vi "Update.vi"(8 "error in (no error)":errorcluster, 10 "Message in":refnum<class "UpdateMessage.lvclass">, 11 "AOTF in":refnum<class "Invivo_AOTF.lvclass">) -> (0 "error out":errorcluster, 3 "AOTF out":refnum<class "Invivo_AOTF.lvclass">)   [LabVIEW 2012, in "Invivo_AOTF.lvclass"]
doc: "The update method processes the command 'update'. \n\nThe command 'update' is used for receiving new values to be set to the private data of the class. This could be seen as a public set method for setting new parameters to the private class data."
uses:
  Invivo_AOTF.lvclass
  <vilib>/Distrio/Murmex/UpdateMessage/UpdateMessage.lvclass
  Invivo_AOTF.lvclass/Invivo_AOTF.ctl
  Controls/laser line enum.ctl
  <vilib>/Distrio/Murmex/Murmex/Murmex.lvclass
panel:
  # "This method is called when the UPDATE\ntrigger is sent. \n\nOverride this method when your component needs to\nrespond to this trigger. \n\nCall parent for proper implementation"
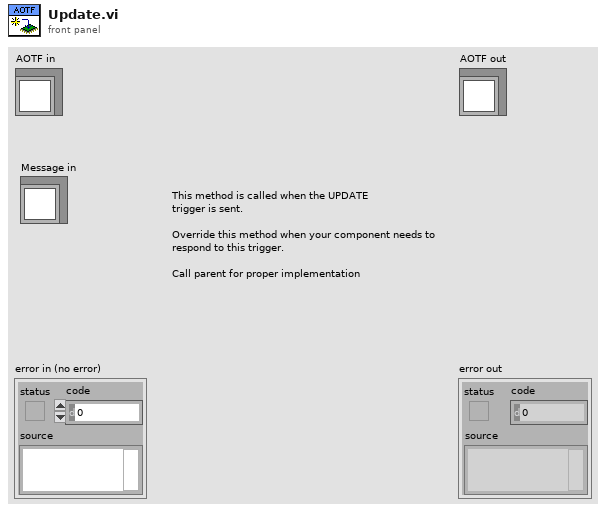
[diagram p1: front panel]
types:
  T1 = typedef "Invivo_AOTF.lvclass/laser line enum.ctl" = dbl
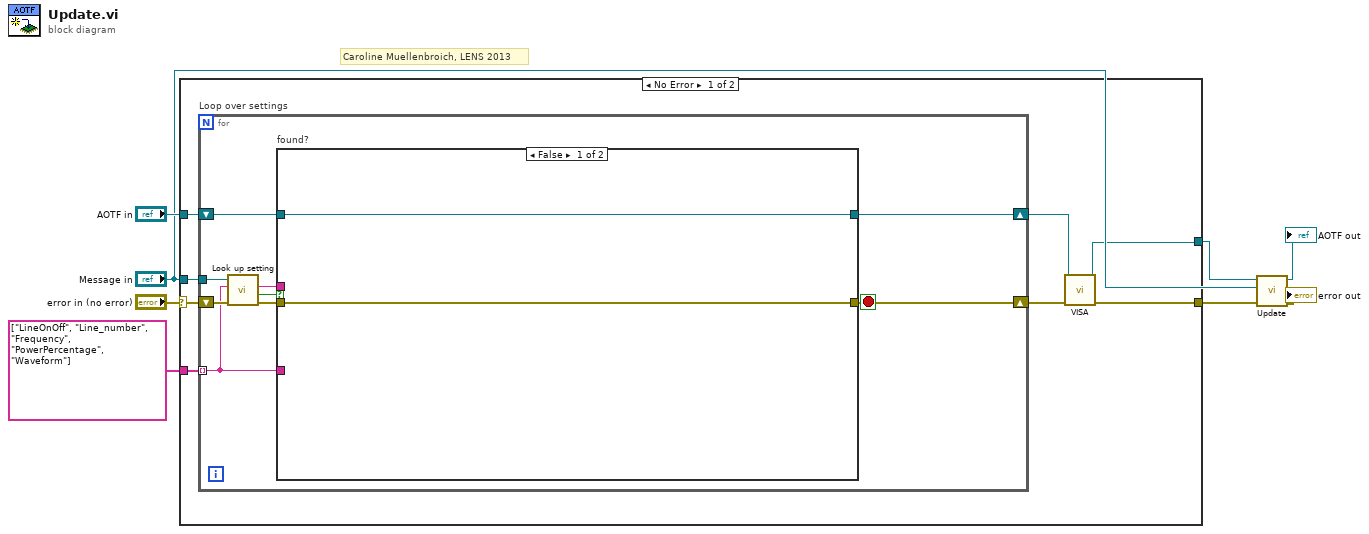
[diagram p0: block diagram]
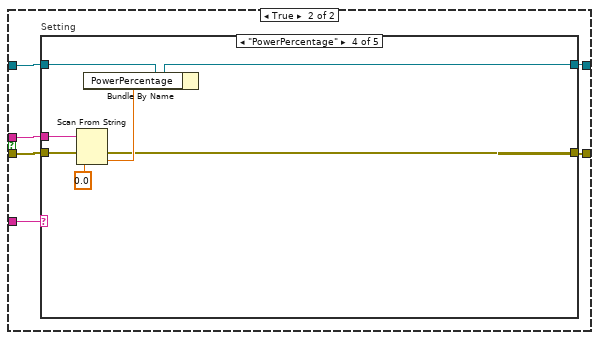
[diagram p2: hidden frame]
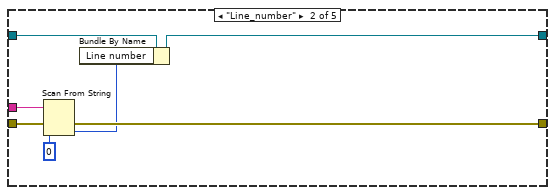
[diagram p4: hidden frame]
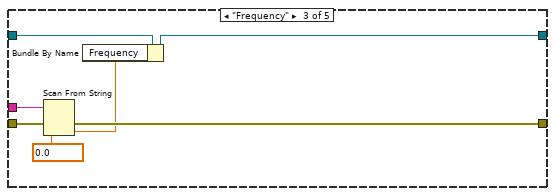
[diagram p5: hidden frame]
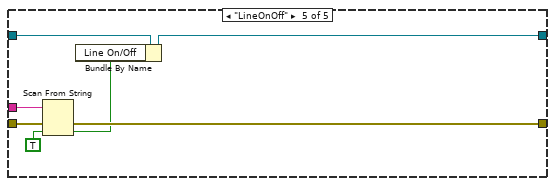
[diagram p6: hidden frame]
diagram:
  # "Caroline Muellenbroich, LENS 2013"
  n1 = case shown="No Error" "error in (no error)" {
    selector: "error in (no error)" -> [w16 w64]
    tunnel: string[] ["LineOnOff", "Line_number", "Frequency", "PowerPercentage", "Waveform"] ("key chains") -> [w15 _]
    tunnel: "Message in" -> [w14 _]
    tunnel: "AOTF in" -> [w13 w65]
    tunnel: [w9 w64] -> w3
    tunnel: [w10 w65] -> w2
    frame No Error {
      n2 = for "Loop over settings" {
        shift-right: [w17] -> w12
        shift-left: w16 -> [w25]
        tunnel: w15 -> [w19] mode=indexing
        tunnel: w14 -> [w24]
        shift-right: [w18] -> w11
        shift-left: w13 -> [w22]
        stop <- w17 stop-if-true
        n3 = call <vilib>:"Look up setting.vi"("error in (no error)"=w25, "tag name"=w19, "UpdateMessage in"=w24) -> ("error out"=w20:errorcluster, "found?"=w23:bool, "value"=w21:string)  [unwired: 5 in, 1 out]
        n4 = case "found?" shown="False" w23 {
          tunnel: w22 -> [w27 w31]
          tunnel: w21 -> [_ w32]
          tunnel: w20 -> [w26 w30]
          tunnel: w19 -> [_ w33]
          tunnel: [w27 w28] -> w18
          tunnel: [w26 w29] -> w17
          frame False {
          }
          frame True {
            n5 = case "Setting" shown="\"PowerPercentage\"" w33 {
              tunnel: w32 -> [_ w36 w48 w50 w59]
              tunnel: w31 -> [w35 w40 w47 w55 w62]
              tunnel: w30 -> [w34 w42 w49 w56 w63]
              tunnel: [w35 w39 w46 w54 w61] -> w28
              tunnel: [w34 w41 w45 w51 w60] -> w29
              frame Default {
              }
              frame "Line_number" {
                n6 = Scan From String(input string=w36, error in=w42, default 1=u32 0 ("Settings_cluster.Line number")) -> (error out=w41:errorcluster, output 1=w38:u32)  [unwired: 2 in, 2 out]
                n7 = Bundle By Name(cluster=w40, "Line number"=w38) -> (w39:refnum<class "Invivo_AOTF.lvclass">)
              }
              frame "Frequency" {
                w44 = T1 0.0 items=["Empty", "445nm (127.4MHz)"] ("Settings cluster.Frequency")
                n8 = Scan From String(input string=w48, error in=w49, default 1=w44) -> (error out=w45:errorcluster, output 1=w43:T1)  [unwired: 2 in, 2 out]
                n9 = Bundle By Name(cluster=w47, "Frequency"=w43) -> (w46:refnum<class "Invivo_AOTF.lvclass">)
              }
              frame "PowerPercentage" {
                n10 = Scan From String(input string=w50, error in=w56, default 1=0.0 ("Settings_cluster.Power")) -> (error out=w51:errorcluster, output 1=w52:dbl)  [unwired: 2 in, 2 out]
                n11 = Bundle By Name(cluster=w55, "PowerPercentage"=w52) -> (w54:refnum<class "Invivo_AOTF.lvclass">)
              }
              frame "LineOnOff" {
                n12 = Scan From String(input string=w59, error in=w63, default 1=TRUE) -> (error out=w60:errorcluster, output 1=w57:bool)  [unwired: 2 in, 2 out]
                n13 = Bundle By Name(cluster=w62, "Line On/Off"=w57) -> (w61:refnum<class "Invivo_AOTF.lvclass">)
              }
            }
          }
        }
      }
      n14 = call-dynamic "VISA.vi"("error in (no error)"=w12, "AOTF in"=w11) -> ("error out"=w9:errorcluster, "AOTF out"=w10:refnum<class "Invivo_AOTF.lvclass">)  [unwired: 8 in]
    }
    frame Error {
    }
  }
  n15 = call-parent "Update.vi"("error in (no error)"=w3, "Message in"="Message in", "Murmex in"=w2) -> ("error out"=→"error out":errorcluster, "Murmex out"=→"AOTF out":refnum<class "Invivo_AOTF.lvclass">)  [unwired: 7 in]
